vi "READ.vi"(11 "TCP Connection Refnum in":refnum<k5>) -> (3 "Registers":u16[](array[numeric]))   [LabVIEW 2012]
uses:
  MB Ethernet Master Query Folder/NI Modbus.llb/MB Modbus Command.ctl
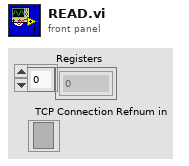
[diagram p1: front panel]
types:
  T1 = typedef "MB Modbus Command.ctl" = cluster{"Function Code":u8, "Starting Address":u16, "Quantity":u16, "Data":u16[], "Discrete":bool[]}
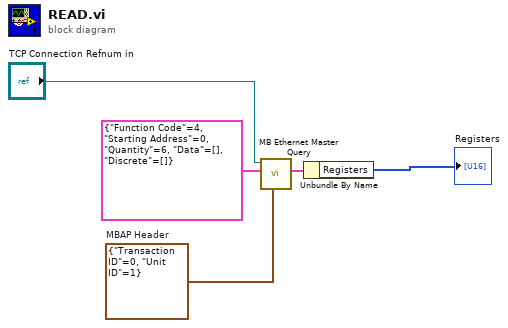
[diagram p0: block diagram]
diagram:
  w3 = cluster{"Transaction ID":u16, "Unit ID":u8} {"Transaction ID"=0, "Unit ID"=1}  # MBAP Header
  n1 = call "MB Ethernet Master Query.vi"("MBAP Header"=w3, "Modbus Command"=T1 {"Function Code"=4, "Starting Address"=0, "Quantity"=6, "Data"=[], "Discrete"=[]} ("MODBUS Command"), "TCP Connection Refnum in"="TCP Connection Refnum in") -> ("Registers"=w5:cluster{"Registers":u16[], "Discrete":bool[]})  [unwired: 4 in, 4 out]
  n2 = Unbundle By Name(w5) -> ("Registers"=→"Registers":u16[])
